vi "例5.5“删除数组元素”函数.vi"() -> ()   [LabVIEW 2017]
panel:
  out "结果":i32[](array[numeric])
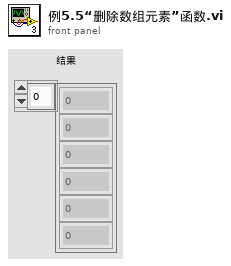
[diagram p1: front panel]
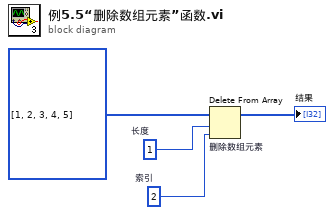
[diagram p0: block diagram]
diagram:
  w2 = 2  # 索引
  w3 = 1  # 长度
  n1 = Delete From Array "删除数组元素"(array=i32[] [1, 2, 3, 4, 5], length=w3, index=w2) -> (array with subset deleted=→"结果":i32[])  [unwired: 1 out]
